vi "Begin.vi"(8 "error in":errorcluster) -> (0 "error out":errorcluster)   [LabVIEW 2017]
doc: "Called before other user functions, this VI is expected to open initial I/O refnums, load in file data, and do all program initialization. Notice that the <B>error out</B> terminal is simply used for data flow. Wiring it to other structures or subVIs ensures that this VI runs first."
uses:
  <vilib>/Rock Robotics/WPI/DriverStation/WPI_DriverStationRobotMode2.ctl
  CommandTypes/ClimbCommands.ctl
  CommandTypes/DriveCommands.ctl
  CommandTypes/LiftCommands.ctl
  CommandTypes/IntakeCommands.ctl
  <vilib>/Rock Robotics/SystemInterfaces/i2clib/i2c_bus.ctl
  <vilib>/Rock Robotics/SystemInterfaces/DIO/FPGA_DIOChannel.ctl
  <vilib>/Rock Robotics/WPI/Joystick/WPI_JoystickDeviceEnum.ctl
  <vilib>/Rock Robotics/SystemInterfaces/DIO/FPGA_DIOPWMChannel.ctl
  <vilib>/Rock Robotics/WPI/ThirdParty/Phoenix-LabVIEW/Motor Controller/Controls/CTRE_Phoenix_MotorControl_FeedbackDevice.ctl
  <userlib>/836-Library/System/QCP_V2/QCPSupportCode/QCPData.ctl
  <userlib>/836-Library/Drive/Drive_Code_V2/Drive_Code_Support/SensorTypedefs/Sensor_Cluster.ctl
  <userlib>/836-Library/Drive/Drive_Code_V2/Drive_Code_Support/SensorTypedefs/Camera_Cluster.ctl
  <vilib>/Rock Robotics/WPI/RobotDrive/WPI_RobotDriveDevRef.ctl
  <vilib>/Rock Robotics/WPI/MotorControl/WPI_MotorControlDeviceRef.ctl
  <vilib>/Rock Robotics/WPI/MotorControl/WPI_MotorControlType.ctl
  <vilib>/Rock Robotics/WPI/PWM/WPI_PWMDeadband.ctl
  <userlib>/836-Library/Drive/Drive_Code_V2/Drive_Code_Support/DriveTrains/Drive_Trains.ctl
  <userlib>/836-Library/Drive/Drive_Code_V2/Drive_Code_Support/Command_Sends/Drive_Code_Command_Type.ctl
  <userlib>/836-Library/Drive/Drive_Code_V2/Drive_Code_Support/Command_Sends/Drive_Code_Command_List.ctl
  <userlib>/836-Library/Drive/Drive_Code_V2/Drive_Code_Support/PidClusters/PidInversions.ctl
  <userlib>/836-Library/Drive/Drive_Code_V2/Drive_Code_Support/PidClusters/DrivePidInputs.ctl
  <userlib>/836-Library/Drive/Drive_Code_V2/Drive_Code_Support/PidClusters/PidInputs.ctl
  <userlib>/836-Library/Drive/Drive_Code_V2/Drive_Code_Support/Command_Sends/Command_Tolerances.ctl
  <userlib>/836-Library/Drive/Drive_Code_V2/Drive_Code_Support/Command_Sends/Command_Tolerance_Info.ctl
  Robot Global Data.vi
  <userlib>/836-Library/Drive/Drive_Code_V2/Drive_Code_Support/DriveTrains/Tank/Tank_6_Motor.vi
  <vilib>/Rock Robotics/WPI/Counter/WPI_CounterDigitalInputToDigitalSource.vi
  <vilib>/Rock Robotics/WPI/MotorControl/WPI_MotorControlOpen Talon.vi
  SharedVarLibs/Notifiers.lvlib
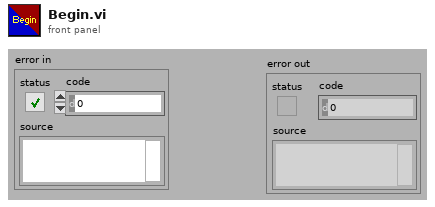
[diagram p1: front panel]
types:
  T1 = typedef "CTRE_Phoenix_MotorControl_FeedbackDevice.ctl" = i8
  T2 = typedef "FPGA_DIOChannel.ctl" = enum8{"DIO 0", "DIO 1", "DIO 2", "DIO 3", "DIO 4", "DIO 5", "DIO 6", "DIO 7", "DIO 8", "DIO 9", "DIO MXP 0", "DIO MXP 1", "DIO MXP 2", "DIO MXP 3", "DIO MXP 4", "DIO MXP 5", "DIO MXP 6", "DIO MXP 7", "DIO MXP 8", "DIO MXP 9", "DIO MXP 10", "DIO MXP 11", "DIO MXP 12", "DIO MXP 13", "DIO MXP 14", "DIO MXP 15", "SPI Port CS1", "SPI Port CS2", "SPI Port CS3", "SPI Port MISO", "SPI Port MOSI", "Invalid"}
  T3 = typedef "FPGA_DIOPWMChannel.ctl" = enum8{"PWM 0", "PWM 1", "PWM 2", "PWM 3", "PWM 4", "PWM 5", "PWM 6", "PWM 7", "PWM 8", "PWM 9", "PWM MXP 0", "PWM MXP 1", "PWM MXP 2", "PWM MXP 3", "PWM MXP 4", "PWM MXP 5", "PWM MXP 6", "PWM MXP 7", "PWM MXP 8", "PWM MXP 9", "Invalid"}
  T4 = typedef "WPI_JoystickDeviceEnum.ctl" = enum16{"USB 0", "USB 1", "USB 2", "USB 3", "USB 4", "USB 5"}
  T5 = typedef "i2c_bus.ctl" = enum16{"I2C On-Board", "I2C MXP", "Invalid"}
  T6 = enum32{"P0", "P1", "P2", "P3", "P4", "P5", "P6", "P7"}
  T7 = enum8{"ConfigMode", "AccOnly", "MagOnly", "GyroOnly", "AccMag", "AccGyro", "MagGyro", "AMG", "IMU", "Compass", "M4G", "NDOF_FMC_OFF", "NDOF"}
  T8 = typedef "Notifiers.lvlib/IntakeCommands.ctl" = enum16{"Do Nothing", "Manuel", "Score", "Acquire"}
  T9 = typedef "Notifiers.lvlib/LiftCommands.ctl" = enum16{"Do  Nothing", "Manuel", "Zero", "Ground", "To Switch", "To Scale Low", "To Scale Medium", "To Scale High"}
  T10 = typedef "Notifiers.lvlib/DriveCommands.ctl" = enum16{"Center on Cube", "Manual", "Acquire Cube", "Drive Path"}
  T11 = typedef "Notifiers.lvlib/ClimbCommands.ctl" = enum16{"Do Nothing", "Deploy", "Lift bot"}
  T12 = typedef "WPI_DriverStationRobotMode2.ctl" = enum16{"Autonomous Disabled", "Autonomous Enabled", "Teleop Disabled", "Teleop Enabled", "Disconnected", "Finish", "Test Disabled", "Test Enabled", "Emergency Stopped"}
  T13 = typedef "WPI_MotorControlDeviceRef.ctl" = cluster{"DeviceStatus":errorcluster, "Type":T14, "PWM":cluster{"PWM Channel":T3, "DeadBand":T15}, "CAN":cluster{"Device Number":u8, "SetOutput VI Ref":variant, "GetOutput VI Ref":variant, "Enable VI Ref":variant, "Disable VI Ref":variant, "Data":variant}, "Invert":bool, "DIO PWM":cluster{"PWM \"Enable\" Channel":T3, "DIOChannel":T2, "PWM Rate":dbl}}
  T14 = typedef "WPI_MotorControlType.ctl" = enum16{"PWM", "CAN", "DIO PWM"}
  T15 = typedef "WPI_PWMDeadband.ctl" = cluster{"Name":string, "maxPositivePwm":i32, "minPositivePwm":i32, "centerPwm":i32, "maxNegativePwm":i32, "minNegativePwm":i32, "angularRange":u16}
  T16 = typedef "Drive_Code_Bundle.ctl" = cluster{"Sensor Data":T17, "RobotDriveDevRef":T19, "Drive Train":T20, "Valid Commands":bool[], "Drive Comand Notifier":refnum<notifier>, "Command Finished?":refnum<k4>, "Command Canceled":refnum<k4>, "PID Inversions":T21, "PID Inputs Notifier":refnum<notifier>, "Cmd Tol Notifier":refnum<notifier>}
  T17 = typedef "Sensor_Cluster.ctl" = cluster{"Gyro Data":cluster{"Gyro RT FIFO":refnum<k33>, "Gyro Current":dbl, "Gyro Hold":dbl}, "Encoder Data":cluster{"Encoder RT FIFO":refnum<k33>, "Encoder Current":dbl, "Encoder Hold":dbl}, "Camera Data":cluster{"Camera RT FIFO":refnum<k33>, "Camera Current":T18}}
  T18 = typedef "Camera_Cluster.ctl" = cluster{" Angle":dbl, "Valid":bool}
  T19 = typedef "WPI_RobotDriveDevRef.ctl" = cluster{"DevStatus":errorcluster, "Motors[]":T13[], "Square Inputs":bool, "Max Output":dbl}
  T20 = typedef "Drive_Trains.ctl" = enum16{"Tank Drive 2 Motor", "Tank Drive 4 Motor", "Tank Drive 6 Motor", "Mecanum Drive", "Kiwi Drive", "Invalid"}
  T21 = typedef "PidInversions.ctl" = cluster{"Distance PID Inverted?":bool, "Yaw PID Inverted?":bool}
  T22 = typedef "WPI_DigitalInputDevRef.ctl" = cluster{"DevStatus":errorcluster, "DIO Channel":T2}
  T23 = typedef "FPGA_CounterEncoderSourceConvertionLVSourceType.ctl" = cluster{"DevStatus":errorcluster, "AnalogTriggerMode?":bool, "DigitalMode":cluster{"DIO Channel":T24}, "AnalogTriggerMode":cluster{"AnalogTriggerIndex":T25, "OutputType":T26}}
  T24 = typedef "FPGA_DIODigitalSourceChannel.ctl" = enum8{"DIO 0", "DIO 1", "DIO 2", "DIO 3", "DIO 4", "DIO 5", "DIO 6", "DIO 7", "DIO 8", "DIO 9", "DIO MXP 0", "DIO MXP 1", "DIO MXP 2", "DIO MXP 3", "DIO MXP 4", "DIO MXP 5", "DIO MXP 6", "DIO MXP 7", "DIO MXP 8", "DIO MXP 9", "DIO MXP 10", "DIO MXP 11", "DIO MXP 12", "DIO MXP 13", "DIO MXP 14", "DIO MXP 15", "Disabled"}
  T25 = typedef "FPGA_AnalogTriggerIndex.ctl" = enum8{"Trig 0", "Trig 1", "Trig 2", "Trig 3", "Trig 4", "Trig 5", "Trig 6", "Trig 7", "Invalid"}
  T26 = typedef "FPGA_AnalogTriggerOutType.ctl" = enum16{"InWindow", "TriggerState", "Rising", "Falling"}
  T27 = typedef "WPI_EncoderDevRef.ctl" = cluster{"DevStatus":errorcluster, "EncoderIndex":T28, "CounterIndex":T29, "DistancePerCount":dbl, "Decoding Type":T30}
  T28 = typedef "FPGA_EncoderIdx.ctl" = enum8{"Enc 0", "Enc 1", "Enc 2", "Enc 3", "Enc 4", "Enc 5", "Enc 6", "Enc 7", "Invalid"}
  T29 = typedef "FPGA_CounterCtrSystemIndex.ctl" = enum8{"Ctr 0", "Ctr 1", "Ctr 2", "Ctr 3", "Ctr 4", "Ctr 5", "Ctr 6", "Ctr 7", "Invalid"}
  T30 = typedef "WPI_EncoderType.ctl" = enum16{"1x", "2x", "4x"}
  T31 = typedef "QCP_RefNum.ctl" = cluster{"Data Value Refnum":refnum<data-value>, "semaphore":T32}
  T32 = typedef "Semaphore RefNum" = refnum<k1>
  T33 = typedef "ImuDevRef.ctl" = cluster{"I2CDevRef":T34, "Valid Cal File?":bool}
  T34 = typedef "WPI_I2CDevRef.ctl" = cluster{"DevStatus":errorcluster, "Device Address":u8, "Handle":i32, "I2C Bus":T5}
  T35 = typedef "WPI_JoystickDevRef.ctl" = cluster{"Device":T4}
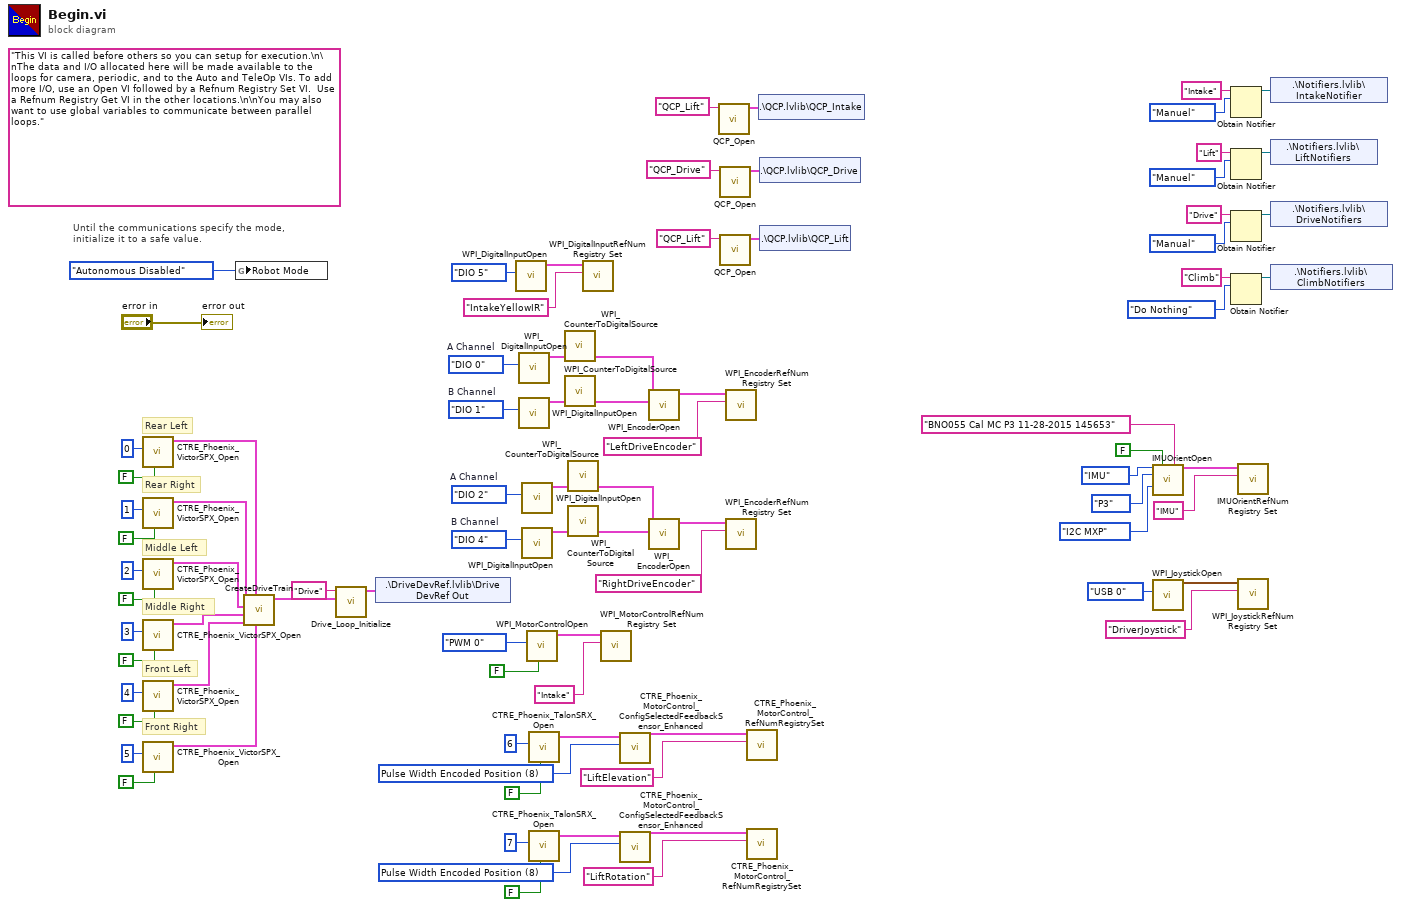
[diagram p0: block diagram]
diagram:
  w10 = T1 8 items=["None"=-1, "QuadEncoder"=0, "Analog"=2, "Tachometer"=4, "Pulse Width Encoded Position"=8, "Sensor Sum (S0 + S1)"=9, "Sensor Difference (D0 - D1)"=10, "Remote Source 0"=11, "Remote Source 1"=12, "Software Emulated"=15] ("Feedback Device")
  w16 = T1 8 items=["None"=-1, "QuadEncoder"=0, "Analog"=2, "Tachometer"=4, "Pulse Width Encoded Position"=8, "Sensor Sum (S0 + S1)"=9, "Sensor Difference (D0 - D1)"=10, "Remote Source 0"=11, "Remote Source 1"=12, "Software Emulated"=15] ("Feedback Device")
  w37 = FPGA_DIOChannel."DIO 4"  # B Channel
  w36 = FPGA_DIOChannel."DIO 2"  # A Channel
  w45 = FPGA_DIOChannel."DIO 1"  # B Channel
  w44 = FPGA_DIOChannel."DIO 0"  # A Channel
  (unwired) "This VI is called before others so you can setup for execution.\n\nThe data and I/O allocated here will be made available to the loops for camera, periodic, and to the Auto and TeleOp VIs. To add more I/O, use an Open VI followed by a Refnum Registry Set VI.  Use a Refnum Registry Get VI in the other locations.\n\nYou may also want to use global variables to communicate between parallel loops."
  # "Front Right"
  # "Front Left"
  # "Middle Right"
  # "Middle Left"
  # "Rear Right"
  # "Rear Left"
  # "Until the communications specify the mode,\ninitialize it to a safe value."
  n1 = call <vilib>:"CTRE_Phoenix_VictorSPX_Open.vi"("Invert"=FALSE, "Device Number"=u8 0) -> ("CAN Talon SRX Ref"=w70:T13)  [unwired: 8 in, 1 out]
  n2 = call <vilib>:"CTRE_Phoenix_VictorSPX_Open.vi"("Invert"=FALSE, "Device Number"=u8 1) -> ("CAN Talon SRX Ref"=w69:T13)  [unwired: 8 in, 1 out]
  n3 = call <vilib>:"CTRE_Phoenix_VictorSPX_Open.vi"("Invert"=FALSE, "Device Number"=u8 2) -> ("CAN Talon SRX Ref"=w65:T13)  [unwired: 8 in, 1 out]
  n4 = call <vilib>:"CTRE_Phoenix_VictorSPX_Open.vi"("Invert"=FALSE, "Device Number"=u8 3) -> ("CAN Talon SRX Ref"=w66:T13)  [unwired: 8 in, 1 out]
  n5 = call <vilib>:"CTRE_Phoenix_VictorSPX_Open.vi"("Invert"=FALSE, "Device Number"=u8 4) -> ("CAN Talon SRX Ref"=w67:T13)  [unwired: 8 in, 1 out]
  n6 = call <vilib>:"CTRE_Phoenix_VictorSPX_Open.vi"("Invert"=FALSE, "Device Number"=u8 5) -> ("CAN Talon SRX Ref"=w68:T13)  [unwired: 8 in, 1 out]
  n7 = global write "Robot Global Data.vi" "Robot Mode"(WPI_DriverStationRobotMode2."Autonomous Disabled" ("Robot Mode")) -> ()
  n8 = call-poly <userlib>:"CreateDriveTrain.vi"("Front Right Motor"=w68, "Rear Left Motor"=w70, "Front Left Motor"=w67, "Middle Right Motor"=w66, "Middle Left Motor"=w65, "Rear Right Motor"=w69) -> ("DriveClusterOut"=w72:T16)  [unwired: 5 in]
  n9 = call <userlib>:"Drive_Loop_Initialize.vi"("Drive Train Ref"=w72, "Name"="Drive") -> ("Drive DevRef Out"=w6:T16)  [unwired: 9 in]
  n10 = shared-variable ".\\DriveDevRef.lvlib\\Drive DevRef Out"(w6) -> ()  [unwired: 1 in, 1 out]
  n11 = call <vilib>:"WPI_DigitalInputOpen.vi"("DIO Channel"=FPGA_DIOChannel."DIO 5") -> ("DigitalInputDevRef"=w22:T22)  [unwired: 9 in, 1 out]
  n12 = call <vilib>:"WPI_DigitalInputOpen.vi"("DIO Channel"=w44) -> ("DigitalInputDevRef"=w41:T22)  [unwired: 1 in, 9 out]
  n13 = call <vilib>:"WPI_DigitalInputOpen.vi"("DIO Channel"=w45) -> ("DigitalInputDevRef"=w42:T22)  [unwired: 1 in, 9 out]
  n14 = call <vilib>:"WPI_DigitalInputOpen.vi"("DIO Channel"=w36) -> ("DigitalInputDevRef"=w33:T22)  [unwired: 1 in, 9 out]
  n15 = call <vilib>:"WPI_DigitalInputOpen.vi"("DIO Channel"=w37) -> ("DigitalInputDevRef"=w34:T22)  [unwired: 1 in, 9 out]
  n16 = call-poly <vilib>:"WPI_MotorControlOpen.vi"("Invert"=FALSE, "PWM Channel"=FPGA_DIOPWMChannel."PWM 0") -> ("MotorControlDeviceRef"=w24:T13)  [unwired: 8 in, 1 out]
  n17 = call <vilib>:"CTRE_Phoenix_TalonSRX_Open.vi"("Invert"=FALSE, "Device Number"=u8 6) -> ("CAN Talon SRX Ref"=w15:T13)  [unwired: 8 in, 1 out]
  n18 = call <vilib>:"CTRE_Phoenix_TalonSRX_Open.vi"("Invert"=FALSE, "Device Number"=u8 7) -> ("CAN Talon SRX Ref"=w9:T13)  [unwired: 8 in, 1 out]
  n19 = call-poly <vilib>:"WPI_CounterToDigitalSource.vi"("DigitalInputDevRef"=w41) -> ("Digital Source"=w40:T23)  [unwired: 6 out]
  n20 = call-poly <vilib>:"WPI_CounterToDigitalSource.vi"("DigitalInputDevRef"=w42) -> ("Digital Source"=w43:T23)  [unwired: 6 out]
  n21 = call-poly <vilib>:"WPI_CounterToDigitalSource.vi"("DigitalInputDevRef"=w33) -> ("Digital Source"=w32:T23)  [unwired: 6 out]
  n22 = call-poly <vilib>:"WPI_CounterToDigitalSource.vi"("DigitalInputDevRef"=w34) -> ("Digital Source"=w35:T23)  [unwired: 6 out]
  n23 = call <vilib>:"WPI_DigitalInputRefNum Registry Set.vi"("refnum name"="IntakeYellowIR", "DigitalInputDevRef"=w22) -> ()  [unwired: 8 in, 2 out]
  n24 = call <vilib>:"WPI_MotorControlRefNum Registry Set.vi"("refnum name"="Intake", "MotorControlDevRef"=w24) -> ()  [unwired: 8 in, 2 out]
  n25 = call <vilib>:"CTRE_Phoenix_MotorControl_ConfigSelectedFeedbackSensor_Enhanced.vi"("Feedback Device"=w16, "PhoenixMotorControlDevRef"=w15) -> ("PhoenixMotorControlDevRef"=w14:T13)  [unwired: 8 in, 1 out]
  n26 = call <vilib>:"CTRE_Phoenix_MotorControl_ConfigSelectedFeedbackSensor_Enhanced.vi"("Feedback Device"=w10, "PhoenixMotorControlDevRef"=w9) -> ("PhoenixMotorControlDevRef"=w8:T13)  [unwired: 8 in, 1 out]
  n27 = call <vilib>:"WPI_EncoderOpen.vi"("BSource"=w43, "ASource"=w40) -> ("EncoderDevRef"=w39:T27)  [unwired: 6 in, 3 out]
  n28 = call <vilib>:"WPI_EncoderOpen.vi"("BSource"=w35, "ASource"=w32) -> ("EncoderDevRef"=w31:T27)  [unwired: 6 in, 3 out]
  n29 = call <userlib>:"QCP_Open.vi"("Name"="QCP_Lift") -> ("QCP_DevRef_Out"=w1:T31)  [unwired: 9 in, 1 out]
  n30 = call <userlib>:"QCP_Open.vi"("Name"="QCP_Drive") -> ("QCP_DevRef_Out"=w5:T31)  [unwired: 9 in, 1 out]
  n31 = call <userlib>:"QCP_Open.vi"("Name"="QCP_Lift") -> ("QCP_DevRef_Out"=w3:T31)  [unwired: 9 in, 1 out]
  n32 = call <vilib>:"WPI_EncoderRefNum Registry Set.vi"("refnum name"="LeftDriveEncoder", "EncoderDevRef"=w39) -> ()  [unwired: 8 in, 2 out]
  n33 = call <vilib>:"WPI_EncoderRefNum Registry Set.vi"("refnum name"="RightDriveEncoder", "EncoderDevRef"=w31) -> ()  [unwired: 8 in, 2 out]
  n34 = call <vilib>:"CTRE_Phoenix_MotorControl_RefNumRegistrySet.vi"("refnum name"="LiftElevation", "PhoenixMotorControlDevRef"=w14) -> ()  [unwired: 8 in, 2 out]
  n35 = call <vilib>:"CTRE_Phoenix_MotorControl_RefNumRegistrySet.vi"("refnum name"="LiftRotation", "PhoenixMotorControlDevRef"=w8) -> ()  [unwired: 8 in, 2 out]
  n36 = shared-variable ".\\QCP.lvlib\\QCP_Intake"(w1) -> ()  [unwired: 1 in, 1 out]
  n37 = shared-variable ".\\QCP.lvlib\\QCP_Drive"(w5) -> ()  [unwired: 1 in, 1 out]
  n38 = shared-variable ".\\QCP.lvlib\\QCP_Lift"(w3) -> ()  [unwired: 1 in, 1 out]
  n39 = call <userlib>:"IMUOrientOpen.vi"("Op Mode"=T7."IMU", "Calibrate?"=FALSE, "Stored Cal File"="BNO055 Cal MC P3 11-28-2015 145653", "Placement"=T6."P3", "I2C Bus"=i2c_bus."I2C MXP") -> ("IMU Dev Ref"=w52:T33)  [unwired: 4 in, 6 out]
  n40 = call <vilib>:"WPI_JoystickOpen.vi"("JoystickDevice"=WPI_JoystickDeviceEnum."USB 0") -> ("JoystickDevRef"=w29:T35)  [unwired: 10 in]
  n41 = Obtain Notifier(name (unnamed)="Intake", notification data type=IntakeCommands."Manuel") -> (notifier out=w77:refnum<notifier>)  [unwired: 2 in, 2 out]
  n42 = Obtain Notifier(name (unnamed)="Lift", notification data type=LiftCommands."Manuel") -> (notifier out=w76:refnum<notifier>)  [unwired: 2 in, 2 out]
  n43 = Obtain Notifier(name (unnamed)="Drive", notification data type=DriveCommands."Manual") -> (notifier out=w75:refnum<notifier>)  [unwired: 2 in, 2 out]
  n44 = Obtain Notifier(name (unnamed)="Climb", notification data type=ClimbCommands."Do Nothing") -> (notifier out=w74:refnum<notifier>)  [unwired: 2 in, 2 out]
  n45 = call <userlib>:"IMUOrientRefNum Registry Set.vi"("refnum name"="IMU", "IMUDevRef in"=w52) -> ()  [unwired: 8 in, 2 out]
  n46 = call <vilib>:"WPI_JoystickRefNum Registry Set.vi"("refnum name"="DriverJoystick", "JoystickDevRef"=w29) -> ()  [unwired: 8 in, 2 out]
  n47 = shared-variable ".\\Notifiers.lvlib\\IntakeNotifier"(w77) -> ()  [unwired: 1 in, 1 out]
  n48 = shared-variable ".\\Notifiers.lvlib\\LiftNotifiers"(w76) -> ()  [unwired: 1 in, 1 out]
  n49 = shared-variable ".\\Notifiers.lvlib\\DriveNotifiers"(w75) -> ()  [unwired: 1 in, 1 out]
  n50 = shared-variable ".\\Notifiers.lvlib\\ClimbNotifiers"(w74) -> ()  [unwired: 1 in, 1 out]
  "error out" <- "error in"
